vi "Indexing objective waveform with PDF.vi"(0 "AO sampling rate":dbl, 1 "PFI0 digital clock frequency":dbl, 2 "Steps per Volume":dbl, 4 "Time per volume (s)":dbl, 5 "Window size for layer index (ms)":dbl, 8 "Steps Waveform":waveform(dbl) caption="Waveform") -> (7 "Plane Indexing data":bool[](array[boolean]), 9 "size(s)":i32)   [LabVIEW 2018]
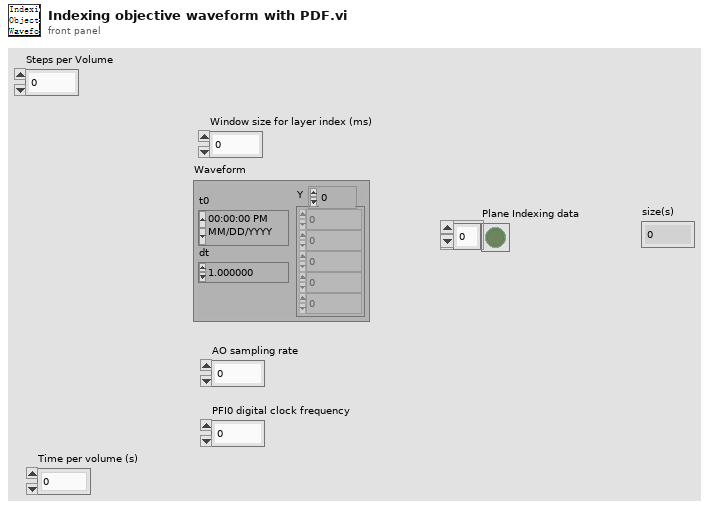
[diagram p1: front panel]
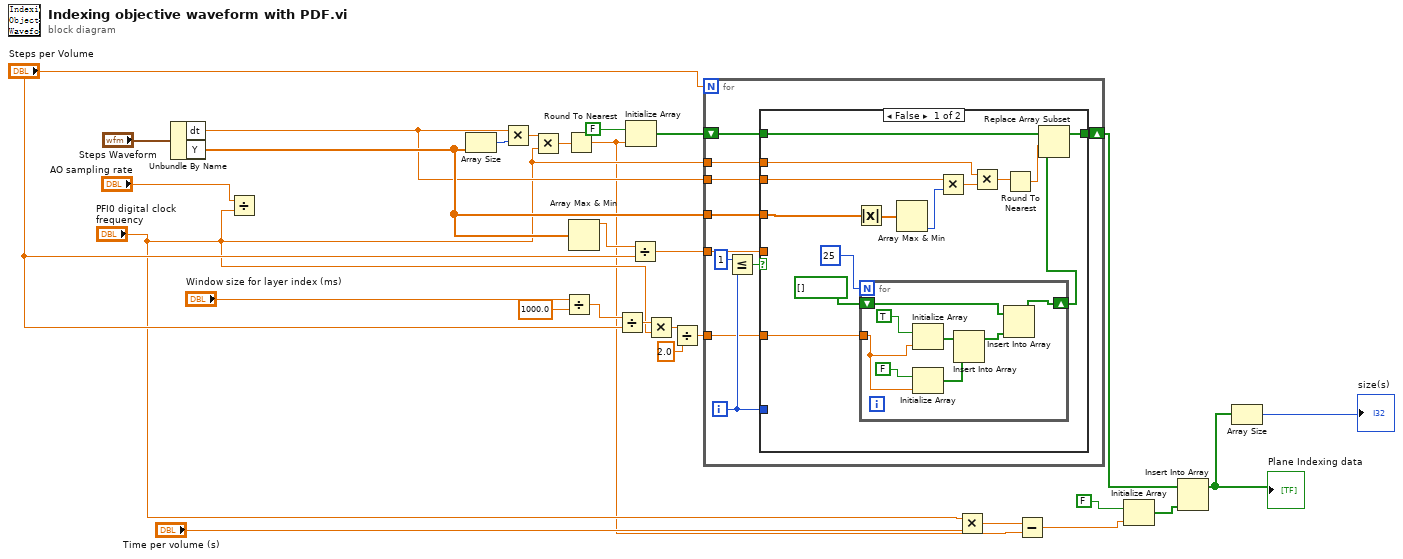
[diagram p0: block diagram]
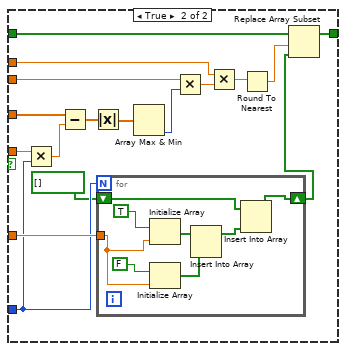
[diagram p2: hidden frame]
diagram:
  n1 = Unbundle By Name("Steps Waveform") -> ("dt"=w3:dbl, "Y"=w4:dbl[])
  n2 = Divide(x="AO sampling rate", y="PFI0 digital clock frequency") -> ()  [unwired: 1 out]
  n3 = Array Size(array=w4) -> (size(s)=w7:i32)
  n4 = Multiply(x=w3, y=w7) -> (x*y=w6:dbl)
  n5 = Multiply(x=w6, y="PFI0 digital clock frequency") -> (x*y=w5:dbl)
  n6 = Divide(x="Window size for layer index (ms)", y=1000.0) -> (x/y=w26:dbl)
  n7 = Round To Nearest(number=w5) -> (nearest integer value=w1:dbl)
  n8 = Array Max & Min(array=w4) -> (max value=w24:dbl)  [unwired: 3 out]
  n9 = Divide(x=w26, y="Steps per Volume") -> (x/y=w20:dbl)
  n10 = Initialize Array(FALSE, w1) -> (w25:bool[])
  n11 = Divide(x=w24, y="Steps per Volume") -> (x/y=w27:dbl)
  n12 = Multiply(x=w20, y="PFI0 digital clock frequency") -> (x*y=w19:dbl)
  n13 = Divide(x=w19, y=2.0) -> (x/y=w17:dbl)
  n14 = for {
    N: "Steps per Volume" -> [_]
    tunnel: w27 -> [w39]
    tunnel: w4 -> [w38]
    shift-right: [w33] -> w12
    shift-left: w25 -> [w37]
    tunnel: w17 -> [w32]
    tunnel: w3 -> [w31]
    tunnel: "PFI0 digital clock frequency" -> [w30]
    i -> [w35]
    n15 = Less Or Equal?(x=1, y=w35) -> (x <= y?=w36:bool)
    n16 = case shown="False" w36 {
      tunnel: w39 -> [_ w78]
      tunnel: w38 -> [w42 w76]
      tunnel: w37 -> [w46 w73]
      tunnel: [w45 w72] -> w33
      tunnel: w35 -> [_ w70]
      tunnel: w32 -> [w40 w71]
      tunnel: w31 -> [w43 w66]
      tunnel: w30 -> [w44 w64]
      frame False {
        n17 = Absolute Value(x=w42) -> (abs(x)=w53:dbl[])
        n18 = for {
          N: 25 -> [_]
          shift-right: [w55] -> w51
          shift-left: bool[] [] -> [w56]
          tunnel: w40 -> [w54]
          n19 = Initialize Array(TRUE, w54) -> (w61:bool[])
          n20 = Initialize Array(FALSE, w54) -> (w60:bool[])
          n21 = Insert Into Array(array=w61, new element=w60) -> (w57:bool[])  [unwired: 1 in]
          n22 = Insert Into Array(array=w56, new element=w57) -> (w55:bool[])  [unwired: 1 in]
        }
        n23 = Array Max & Min(array=w53) -> (min index (indices)=w50:i32)  [unwired: 3 out]
        n24 = Multiply(x=w43, y=w50) -> (x*y=w49:dbl)
        n25 = Multiply(x=w44, y=w49) -> (x*y=w48:dbl)
        n26 = Round To Nearest(number=w48) -> (nearest integer value=w47:dbl)
        n27 = Replace Array Subset(array=w46, new element=w51, index=w47) -> (w45:bool[])
      }
      frame True {
        n28 = Multiply(x=w78, y=w70) -> (x*y=w77:dbl)
        n29 = Subtract(x=w76, y=w77) -> (x-y=w75:dbl[])
        n30 = Absolute Value(x=w75) -> (abs(x)=w74:dbl[])
        n31 = for {
          N: w70 -> [_]
          tunnel: w71 -> [w82]
          shift-right: [w79] -> w68
          shift-left: bool[] [] -> [w80]
          n32 = Initialize Array(TRUE, w82) -> (w86:bool[])
          n33 = Initialize Array(FALSE, w82) -> (w85:bool[])
          n34 = Insert Into Array(array=w86, new element=w85) -> (w81:bool[])  [unwired: 1 in]
          n35 = Insert Into Array(array=w80, new element=w81) -> (w79:bool[])  [unwired: 1 in]
        }
        n36 = Array Max & Min(array=w74) -> (min index (indices)=w67:i32)  [unwired: 3 out]
        n37 = Multiply(x=w66, y=w67) -> (x*y=w65:dbl)
        n38 = Multiply(x=w64, y=w65) -> (x*y=w63:dbl)
        n39 = Round To Nearest(number=w63) -> (nearest integer value=w62:dbl)
        n40 = Replace Array Subset(array=w73, new element=w68, index=w62) -> (w72:bool[])
      }
    }
  }
  n41 = Multiply(x="PFI0 digital clock frequency", y="Time per volume (s)") -> (x*y=w23:dbl)
  n42 = Subtract(x=w23, y=w1) -> (x-y=w16:dbl)
  n43 = Initialize Array(FALSE, w16) -> (w14:bool[])
  n44 = Insert Into Array(array=w12, new element=w14) -> (w9:bool[])  [unwired: 1 in]
  "Plane Indexing data" <- w9
  n45 = Array Size(array=w9) -> (size(s)=→"size(s)":i32)
